vi "Time to subscribe.vi"(8 "error in (no error)":errorcluster, 11 "Measure Object in":refnum<class "Template Module.lvclass">) -> (0 "error out":errorcluster, 3 "Measure Object out":refnum<class "Template Module.lvclass">)   [LabVIEW 2019, in "Template Module.lvclass"]
uses:
  Template Module.lvclass
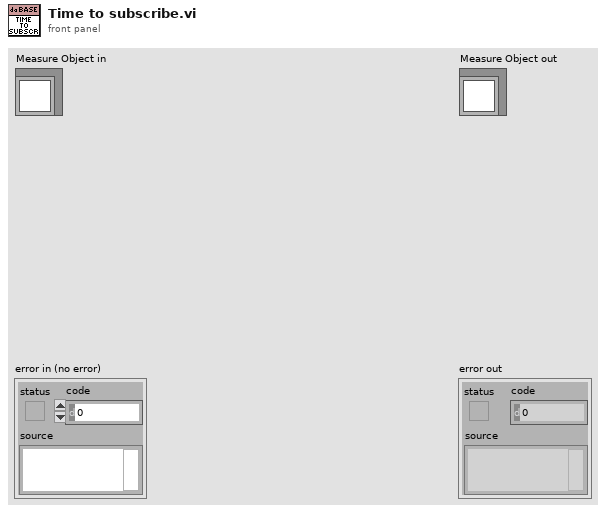
[diagram p1: front panel]
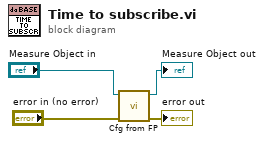
[diagram p0: block diagram]
diagram:
  n1 = call-dynamic "Cfg from FP.vi"("error in (no error)"="error in (no error)", "Measure Object in"="Measure Object in") -> ("error out"=→"error out":errorcluster, "Measure Object out"=→"Measure Object out":refnum<class "Template Module.lvclass">)  [unwired: 8 in]
